vi "example_GInterrupt.vi"() -> ()   [LabVIEW 2020]
uses:
  <vilib>/Galil/resources/gclib/gclib.lvlib
panel:
  out "Interrupt":u8
  out "Error Out":errorcluster
  in  "IP Address":string="192.168.1.77 -s EI --timeout 5000"
  in  "Command":string="EI1; SHA; PA 5000; BGA"
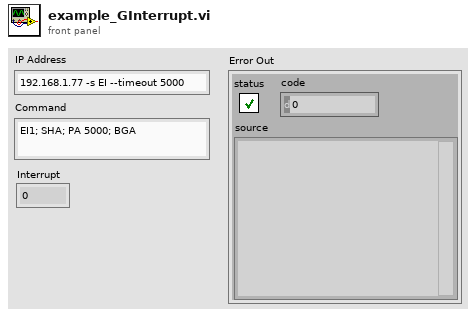
[diagram p1: front panel]
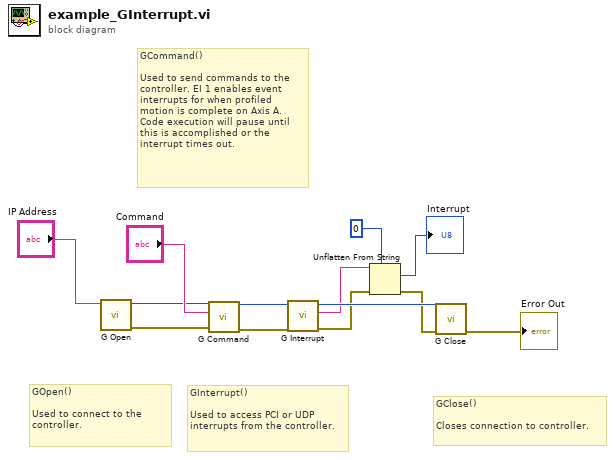
[diagram p0: block diagram]
diagram:
  # "GInterrupt()\n\nUsed to access PCI or UDP interrupts from the controller."
  # "GClose()\n\nCloses connection to controller."
  # "GCommand()\n\nUsed to send commands to the controller. EI 1 enables event interrupts for when profiled motion is complete on Axis A. Code execution will pause until this is accomplished or the interrupt times out."
  # "GOpen()\n\nUsed to connect to the controller."
  n1 = call <vilib>:"G Open.vi"("address"="IP Address") -> ("error out"=w6:errorcluster, "g out"=w7:u64)  [unwired: 8 in]
  n2 = call <vilib>:"G Command.vi"("g"=w7, "command"="Command", "error in (no error)"=w6) -> ("g out"=w10:u64, "error out"=w8:errorcluster)  [unwired: 10 in, 1 out]
  n3 = call <vilib>:"G Interrupt.vi"("error in (no error)"=w8, "g"=w10) -> ("error out"=w4:errorcluster, "status_byte out"=w5:string, "g out"=w9:u64)  [unwired: 7 in]
  n4 = Unflatten From String(type=u8 0, binary string=w5, error in (no error)=w4) -> (value=→"Interrupt":u8, error out=w3:errorcluster)  [unwired: 2 in, 1 out]
  n5 = call <vilib>:"G Close.vi"("error in (no error)"=w3, "g"=w9) -> ("error out"=→"Error Out":errorcluster)  [unwired: 9 in]
